vi "Edit Connector Pane for Wrapper IO Controls.vi"(0 "ControlsIn[]":refnum<vi>[](array[refnum]), 5 "ConPaneIn":refnum<vi>, 11 "error in":errorcluster) -> (4 "OtherControls[]":refnum<vi>[](array[refnum]), 15 "error out":errorcluster)   [LabVIEW 2021, in "Converter.lvlib"]
uses:
  Converter.lvlib
  Converter Reusables/Converter Reusables.lvlib
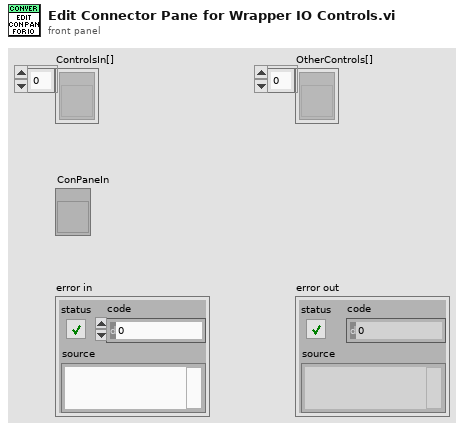
[diagram p1: front panel]
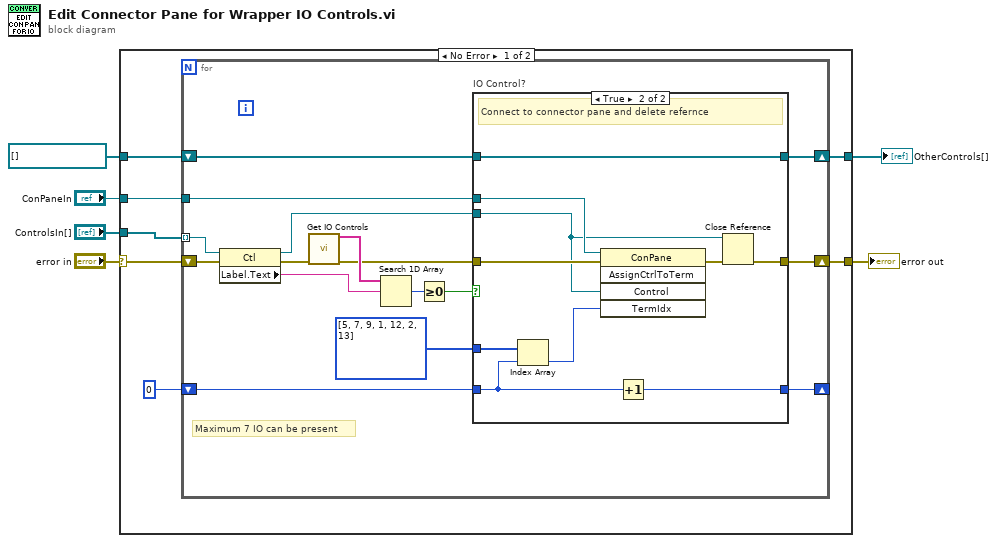
[diagram p0: block diagram]
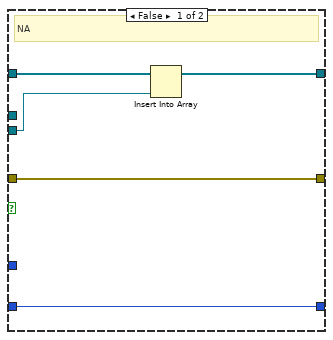
[diagram p2: hidden frame]
diagram:
  n1 = case shown="No Error" "error in" {
    selector: "error in" -> [w10 w46]
    tunnel: "ControlsIn[]" -> [w13 w45]
    tunnel: "ConPaneIn" -> [w11 _]
    tunnel: [w9 w46] -> w3
    tunnel: [w8 w45] -> w2
    tunnel: refnum<vi>[] [] ("ControlsIn[]") -> [w7 _]
    frame No Error {
      n2 = for {
        tunnel: w13 -> [w29] mode=indexing
        shift-right: [w16] -> w8
        shift-left: w7 -> [w17]
        shift-right: [w21] -> _
        shift-left: u32 0 ("Terminal Index") -> [w22]
        tunnel: w11 -> [w19]
        shift-right: [w15] -> w9
        shift-left: w10 -> [w14]
        # "Maximum 7 IO can be present"
        n3 = property class="Ctl"(reference=w29, error in=w14) -> (reference out=w18:refnum<vi>, error out=w28:errorcluster, "Label.Text"=w26:string)
        n4 = call "Get IO Controls.vi"("error in (no error)"=w28) -> ("IO Controls[]"=w27:string[], "error out"=w20:errorcluster)  [unwired: 13 in]
        n5 = Search 1D Array(1D array=w27, element=w26) -> (index of element=w25:i32)  [unwired: 1 in]
        n6 = Greater Or Equal To 0?(x=w25) -> (x >= 0?=w24:bool)
        n7 = case "IO Control?" shown="True" w24 {
          tunnel: u32[] [5, 7, 9, 1, 12, 2, 13] ("Terminal Index") -> [_ w44]
          tunnel: w22 -> [w34 w43]
          tunnel: [w34 w42] -> w21
          tunnel: w20 -> [w33 w41]
          tunnel: w19 -> [_ w40]
          tunnel: w18 -> [w30 w36]
          tunnel: [w33 w37] -> w15
          tunnel: w17 -> [w32 w35]
          tunnel: [w31 w35] -> w16
          frame False {
            # "NA"
            n8 = Insert Into Array(array=w32, new element=w30) -> (w31:refnum<vi>[])  [unwired: 1 in]
          }
          frame True {
            # "Connect to connector pane and delete refernce"
            n9 = Index Array(array=w44, index=w43) -> (element=w39:u32)
            n10 = invoke class="ConPane" method="AssignCtrlToTerm"(reference=w40, error in=w41, "Control"=w36, "TermIdx"=w39) -> (error out=w38:errorcluster)  [unwired: 1 in, 4 out]
            n11 = Increment(x=w43) -> (x+1=w42:u32)
            n12 = Close Reference(reference=w36, error in (no error)=w38) -> (error out=w37:errorcluster)
          }
        }
      }
    }
    frame Error {
    }
  }
  "OtherControls[]" <- w2
  "error out" <- w3
